vi "Copy Template Library.vi"(8 "error in (no error)":errorcluster, 10 "Current Bus Number":i32, 11 "Input Paths":T1) -> (0 "error out":errorcluster, 3 "Current Bus Path":path)   [LabVIEW 2014, in "SPI Engine Scripting.lvlib"]
doc: "Makes a copy of the entire folder/file hierachy of the template library for use by the following scripting steps. The library is named using the current bus number. If there is already a folder with the same name in the desitation directoy, this VI throws an error."
uses:
  SPI Engine Scripting.lvlib
  State Machine/Controls/Input Paths.ctl
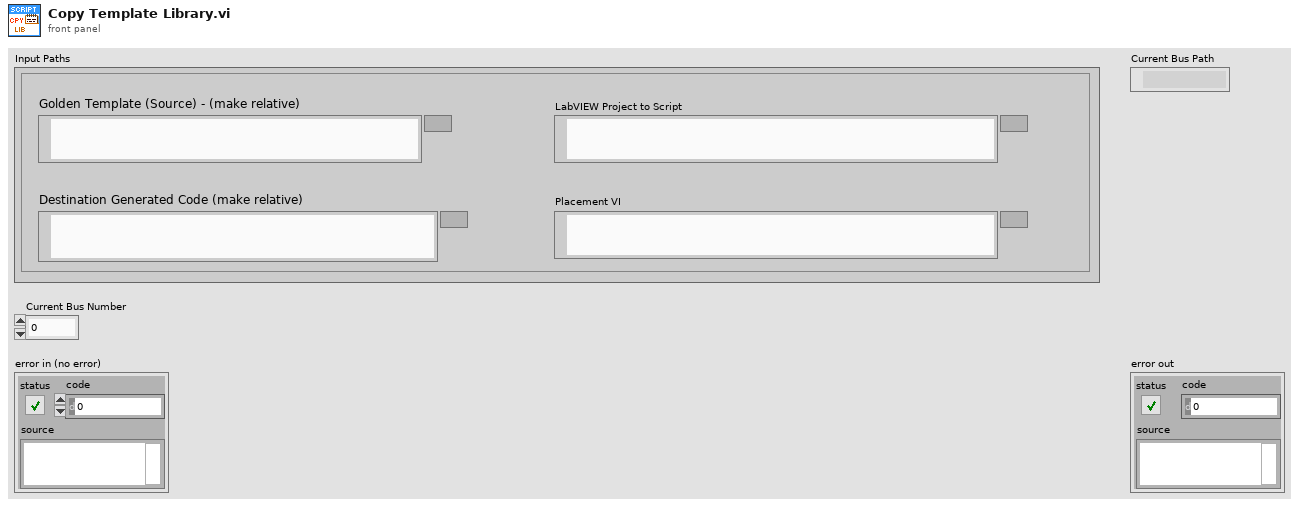
[diagram p1: front panel]
types:
  T1 = typedef "SPI Engine Scripting.lvlib/Input Paths.ctl" = cluster{"Golden Template (Source) - (make relative)":path, "Destination Generated Code (make relative)":path, "LabVIEW Project to Script":path, "Placement VI":path}
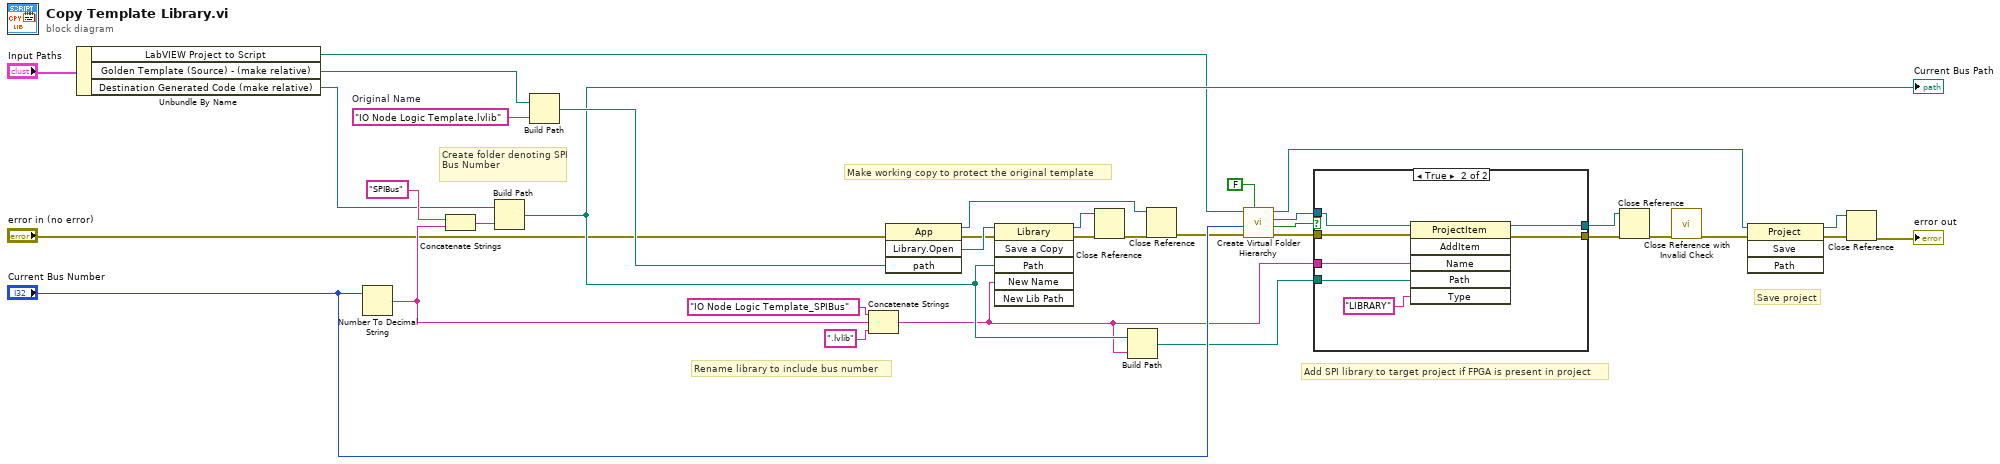
[diagram p0: block diagram]
diagram:
  w33 = "IO Node Logic Template.lvlib"  # Original Name
  # "Add SPI library to target project if FPGA is present in project"
  # "Make working copy to protect the original template"
  # "Save project"
  # "Rename library to include bus number"
  # "Create folder denoting SPI Bus Number"
  n1 = Unbundle By Name("Input Paths") -> ("LabVIEW Project to Script"=w25:path, "Golden Template (Source) - (make relative)"=w30:path, "Destination Generated Code (make relative)"=w31:path)
  n2 = Number To Decimal String(number="Current Bus Number") -> (decimal integer string=w27:string)  [unwired: 1 in]
  n3 = Concatenate Strings("SPIBus" ("string"), w27) -> (w35:string)
  n4 = Build Path(base path=w31, name or relative path=w35) -> (appended path=w28:path)
  "Current Bus Path" <- w28
  n5 = Build Path(base path=w30, name or relative path=w33) -> (appended path=w29:path)
  n6 = Concatenate Strings("IO Node Logic Template_SPIBus" ("string"), w27, ".lvlib" ("string")) -> (w5:string)
  n7 = invoke class="App" method="Library.Open"(error in="error in (no error)", "path"=w29) -> (reference out=w22:refnum<vi>, error out=w18:errorcluster, "Open Library"=w19:refnum<vi>)  [unwired: 2 in, 1 out]
  n8 = invoke class="Library" method="Save a Copy"(reference=w19, error in=w18, "Path"=w28, "New Name"=w5) -> (reference out=w21:refnum<vi>, error out=w20:errorcluster)  [unwired: 2 in, 4 out]
  n9 = Close Reference(reference=w21, error in (no error)=w20) -> (error out=w23:errorcluster)
  n10 = Build Path(base path=w28, name or relative path=w5) -> (appended path=w4:path)
  n11 = Close Reference(reference=w22, error in (no error)=w23) -> (error out=w6:errorcluster)
  n12 = call "Create Virtual Folder Hierarchy.vi"("Create Sub-Bus Folder (F)"=FALSE ("Create Sub-Bus Folder"), "error in"=w6, "Bus Number"="Current Bus Number", "Path to Project"=w25) -> ("error out"=w15:errorcluster, "FPGA Target Found"=w14:bool, "New Virtual Folder"=w13:refnum<vi>, "Project:Open"=w10:refnum<vi>)  [unwired: 4 in]
  n13 = case shown="True" w14 {
    tunnel: w15 -> [w36 w43]
    tunnel: w13 -> [w37 w42]
    tunnel: [w36 w41] -> w9
    tunnel: [w37 w40] -> w8
    tunnel: w5 -> [_ w39]
    tunnel: w4 -> [_ w38]
    frame False {
    }
    frame True {
      n14 = invoke class="ProjectItem" method="AddItem"(reference=w42, error in=w43, "Name"=w39, "Path"=w38, "Type"="LIBRARY") -> (reference out=w40:refnum<vi>, error out=w41:errorcluster)  [unwired: 1 in, 4 out]
    }
  }
  n15 = Close Reference(reference=w8, error in (no error)=w9) -> (error out=w2:errorcluster)
  n16 = call "Close Reference with Invalid Check.vi"("error in (no error)"=w2) -> ("error out"=w1:errorcluster)  [unwired: 10 in]
  n17 = invoke class="Project" method="Save"(reference=w10, error in=w1) -> (reference out=w11:refnum<vi>, error out=w12:errorcluster)  [unwired: 2 in, 2 out]
  n18 = Close Reference(reference=w11, error in (no error)=w12) -> (error out=→"error out":errorcluster)
